vi "ContactCheck.vi"(8 "error in":errorcluster, 11 "task in":refnum<k21>) -> (0 "error out":errorcluster, 3 "Boolesch":bool)   [LabVIEW 2020]
uses:
  <vilib>/DAQmx/read.llb/DAQmx Read (Analog DBL 1Chan 1Samp).vi
  <vilib>/DAQmx/miscellaneous.llb/DAQmx Fill In Error Info.vi
panel:
  out "Waveform Chart":dbl(graph)
  out "data":dbl format="%0.2f"
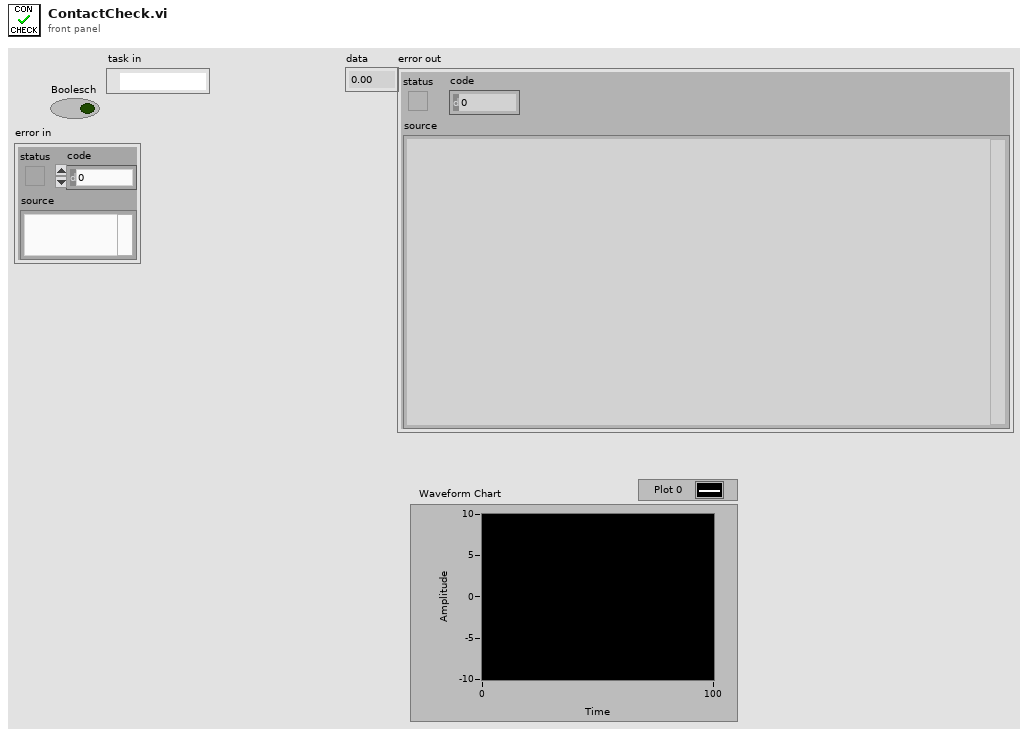
[diagram p1: front panel]
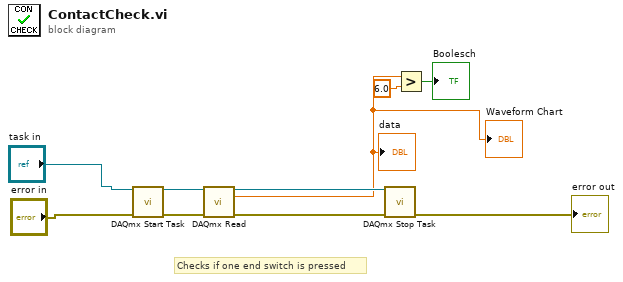
[diagram p0: block diagram]
diagram:
  # "Checks if one end switch is pressed"
  n1 = call <vilib>:"DAQmx Start Task.vi"("task/channels in"="task in", "error in"="error in") -> ("task out"=w9:refnum<k21>, "error out"=w8:errorcluster)  [unwired: 12 in]
  n2 = call-poly <vilib>:"DAQmx Read.vi"("task/channels in"=w9, "error in"=w8) -> ("task out"=w7:refnum<k21>, "data"=w1:dbl, "error out"=w6:errorcluster)  [unwired: 11 in]
  "data" <- w1
  "Waveform Chart" <- w1
  n3 = call <vilib>:"DAQmx Stop Task.vi"("task/channels in"=w7, "error in"=w6) -> ("error out"=→"error out":errorcluster)  [unwired: 12 in, 1 out]
  n4 = Greater?(x=w1, y=6.0) -> (0:→"Boolesch":bool)
